vi "Post Status Update.vi"(8 "error in (no error)":errorcluster, 10 "Cluster":T1, 11 "Asana in":refnum<class "Asana.lvclass">) -> (0 "error out":errorcluster, 2 "gid":string, 3 "Asana out":refnum<class "Asana.lvclass">)   [LabVIEW 2016, in "Asana.lvclass"]
uses:
  levylab_expt_transport/src/Control Experiment/subVIs/Asana/Asana.lvclass
  <vilib>/addons/_JKI.lib/REST Client/classes/REST Client/REST Client.lvclass
  <vilib>/addons/_JKI.lib/Serialization/JSON/JKI JSON Serialization.lvlib
panel:
  out "Response body":string
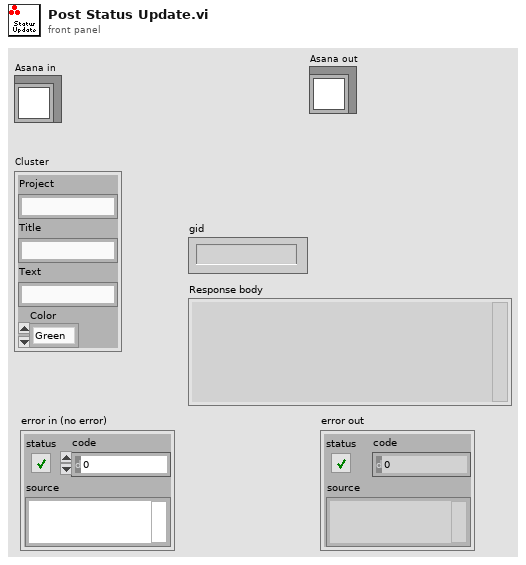
[diagram p1: front panel]
types:
  T1 = cluster{"Project":string, "Title":string, "Text":string, "Color":enum16{"Green", "Yellow", "Red"}}
  T2 = typedef "REST Client.lvlib/REST Client.lvclass/HTTP Header.ctl" = cluster{"header":string, "value":string}
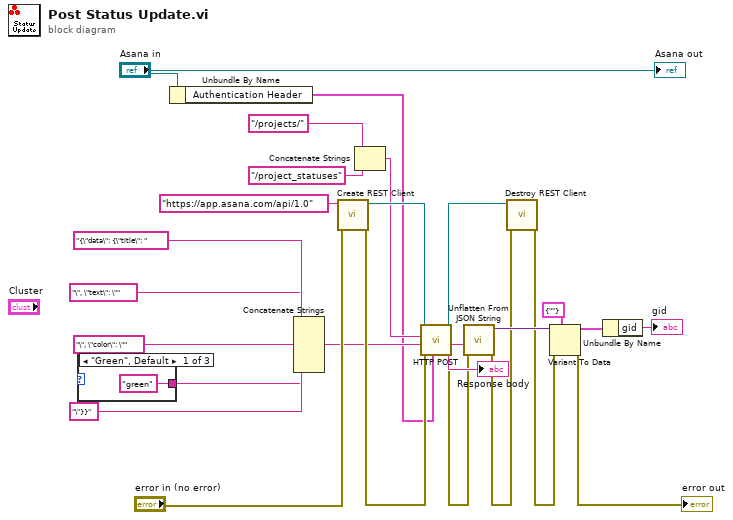
[diagram p0: block diagram]
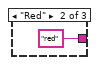
[diagram p2: hidden frame]
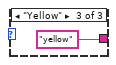
[diagram p3: hidden frame]
diagram:
  n1 = case shown="\"Green\", Default" w4 {
    tunnel: ["green" "red" "yellow"] -> w3
    frame "Green", Default {
    }
    frame "Red" {
    }
    frame "Yellow" {
    }
  }
  n2 = Unbundle By Name("Asana in") -> ("Authentication Header"=w1:T2[])
  n3 = Concatenate Strings("{\"data\": {\"title\": ", "\", \"text\": \"" ("string"), "\", \"color\": \"", w3, "\"}}" ("string")) -> (w24:string, w9:string, w7:string)
  n4 = call <vilib>:"Create REST Client.vi"("error in (no error)"="error in (no error)", "Base URL"="https://app.asana.com/api/1.0") -> ("error out"=w25:errorcluster, "REST Client out"=w28:refnum<class "REST Client.lvclass">)  [unwired: 8 in]
  n5 = Concatenate Strings("/projects/" ("Path"), "/project_statuses") -> (w10:string, w12:string)
  n6 = call-dynamic "HTTP POST.vi"("request specific headers"=w1, "error in (no error)"=w25, "Request body"=w24, "Path"=w10, "REST Client in"=w28) -> ("error out"=w21:errorcluster, "Response body"=w22:string, "REST Client out"=w27:refnum<class "REST Client.lvclass">)  [unwired: 1 in, 3 out]
  "Response body" <- w22
  n7 = call <vilib>:"Unflatten From JSON String.vi"("error in (no error)"=w21, "JSON String"=w22) -> ("error out"=w20:errorcluster, "Variant"=w23:variant)  [unwired: 8 in]
  n8 = call-dynamic "Destroy REST Client.vi"("error in (no error)"=w20, "REST Client in"=w27) -> ("error out"=w19:errorcluster)  [unwired: 9 in]
  n9 = Variant To Data(error in=w19, type=cluster{"gid":string} {"gid"=""}, Variant=w23) -> (data=w16:cluster{"gid":string}, error out=→"error out":errorcluster)
  n10 = Unbundle By Name(w16) -> ("gid"=→"gid":string)
  "Asana out" <- "Asana in"
